vi "CLOSE_WINDOW.vi"(0 "VISA IN":refnum<visa-resource-name>, 5 "error in":errorcluster, 7 "Window":i32) -> (14 "VISA Out":refnum<visa-resource-name>, 19 "error out":errorcluster)   [LabVIEW 2018, in "PNA-X.lvlib"]
doc: "DISPlay:WINDow<wnum>[:STATe] <ON | OFF> \n(Read-Write) Write to create or delete a window on the screen or Read whether a window is present. \nParameters \n<wnum> Window number to create; choose any integer between 1 and the maximum \nnumber of windows allowed in the PNA. \n<ON | OFF> ON (or 1) - The window <wnum> is created. \nOFF (or 0) - The window <wnum> is deleted. \nExamples DISP:WIND ON \ndisplay:window2:state off \nQuery Syntax DISPlay:WINDow<wnum>[:STATe]? \nReturn Type Boolean (1 = ON, 0 = OFF) \nDefault Window number \"1\" ON"
uses:
  PNA-X.lvlib
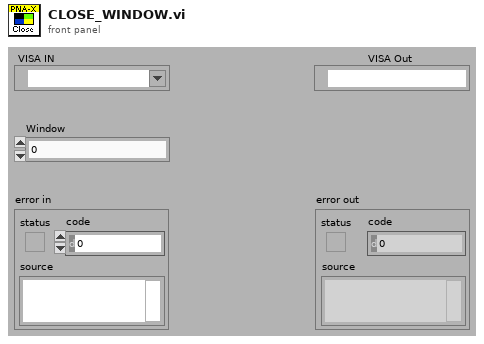
[diagram p1: front panel]
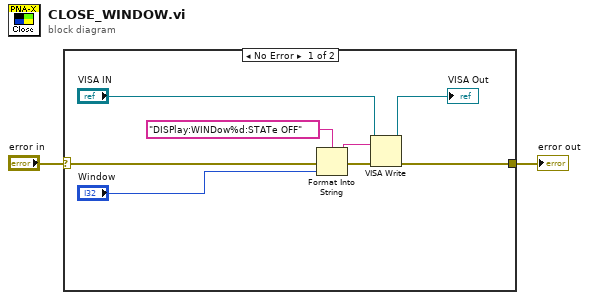
[diagram p0: block diagram]
diagram:
  n1 = case shown="No Error" "error in" {
    selector: "error in" -> [w10 w11]
    tunnel: [w5 w11] -> w1
    frame No Error {
      n2 = Format Into String(format string="DISPlay:WINDow%d:STATe OFF" ("Cmdline"), error in=w10, "Window") -> (resulting string=w8:string, error out=w9:errorcluster)  [unwired: 1 in]
      n3 = VISA Write(VISA resource name="VISA IN", write buffer=w8, error in (no error)=w9) -> (VISA resource name out=→"VISA Out":refnum<visa-resource-name>, error out=w5:errorcluster)  [unwired: 1 out]
    }
    frame Error {
    }
  }
  "error out" <- w1
